vi "UploadFile.vi"(7 "Root Path":path, 8 "error in (no error)":errorcluster, 10 "Path":path, 11 "FTPProtocol in":refnum<class "FTPProtocol.lvclass">) -> (0 "error out":errorcluster, 3 "FTPProtocol out":refnum<class "FTPProtocol.lvclass">)   [LabVIEW 2020, in "FileSync -- FTP.lvlib" / "FTPProtocol.lvclass"]
uses:
  FTPProtocol.lvclass
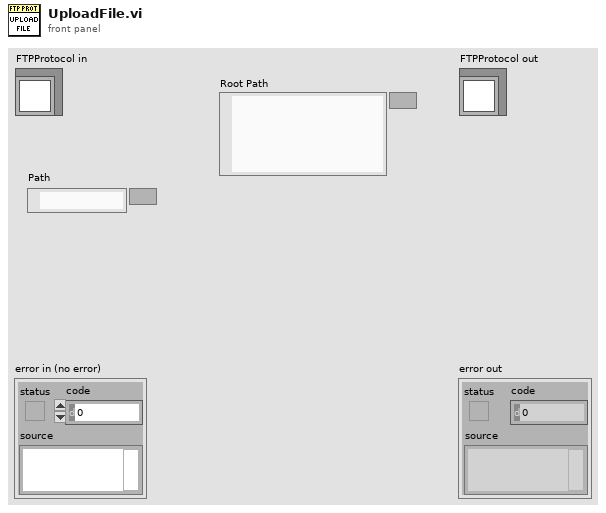
[diagram p1: front panel]
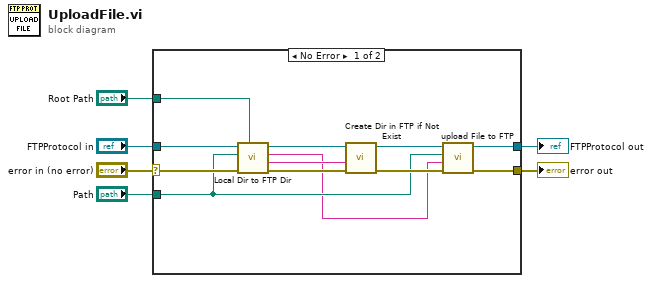
[diagram p0: block diagram]
diagram:
  n1 = case shown="No Error" "error in (no error)" {
    selector: "error in (no error)" -> [w15 w19]
    tunnel: "FTPProtocol in" -> [w17 w20]
    tunnel: "Root Path" -> [w16 _]
    tunnel: [w11 w20] -> w3
    tunnel: [w9 w19] -> w2
    tunnel: "Path" -> [w8 _]
    frame No Error {
      n2 = call "Local Dir to FTP Dir.vi"("Root Path"=w16, "error in (no error)"=w15, "Path"=w8, "FTPProtocol in"=w17) -> ("error out"=w13:errorcluster, "parent folder in ftp"=w14:string, "ftp path"=w7:string, "FTPProtocol out"=w18:refnum<class "FTPProtocol.lvclass">)  [unwired: 4 in]
      n3 = call "Create Dir in FTP if Not Exist.vi"("error in (no error)"=w13, "dir"=w14, "FTPProtocol in"=w18) -> ("error out"=w10:errorcluster, "FTPProtocol out"=w12:refnum<class "FTPProtocol.lvclass">)  [unwired: 7 in]
      n4 = call "upload File to FTP.vi"("error in (no error)"=w10, "ftp path"=w7, "Path"=w8, "FTPProtocol in"=w12) -> ("error out"=w9:errorcluster, "FTPProtocol out"=w11:refnum<class "FTPProtocol.lvclass">)  [unwired: 6 in]
    }
    frame Error {
    }
  }
  "error out" <- w2
  "FTPProtocol out" <- w3
